vi "Get VI Data.vi"(8 "Error In":errorcluster, 10 "Wik Help Base URL":string="https://www.labviewmakerhub.com/doku.php?id=learn:libraries:linx:reference:labview:", 11 "VI Reference":refnum<vi>) -> (0 "Error Out":errorcluster, 3 "VI Data":T1)   [LabVIEW 2014]
uses:
  VI Data.ctl
  Control Info.ctl
  <vilib>/picture/picture.llb/imagedata.ctl
  <vilib>/Utility/traverseref.llb/TRef TravTarget.ctl
  <vilib>/Utility/traverseref.llb/VI Scripting - Traverse.lvlib
  <vilib>/MakerHub/Toolbox/Private/Front Panel Clean Up/LMH-Front-Panel-Clean-Up.lvlib
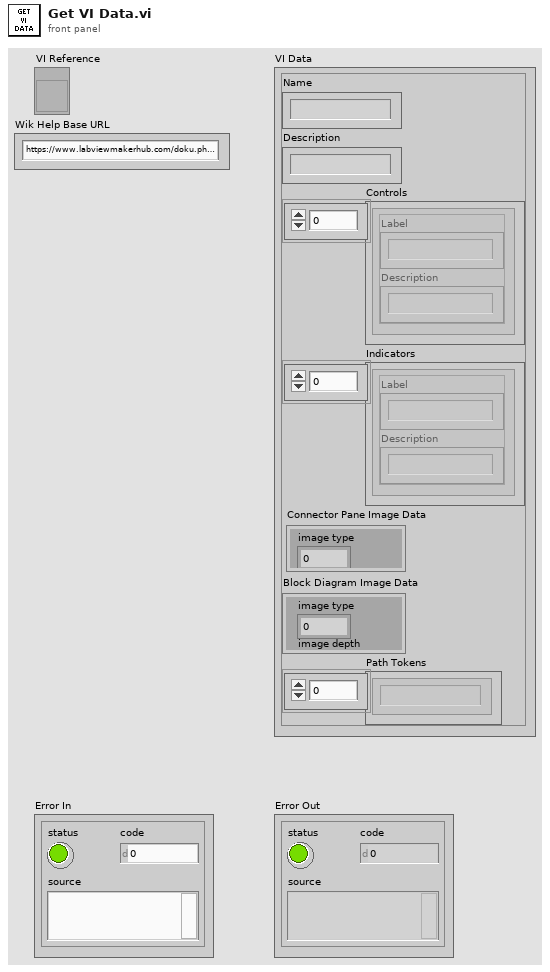
[diagram p1: front panel]
types:
  T1 = typedef "VI Data.ctl" = cluster{"Name":string, "Description":string, "Controls":T2[], "Indicators":T2[], "Connector Pane Image Data":T3, "Block Diagram Image Data":T3, "Path Tokens":string[]}
  T2 = typedef "Control Info.ctl" = cluster{"Label":string, "Description":string}
  T3 = typedef "imagedata.ctl" = cluster{"image type":i32, "image depth":i32, "image":u8[], "mask":u8[], "colors":u32[], "Rectangle":cluster{"left":i16, "top":i16, "right":i16, "bottom":i16}}
  T4 = enum32{"Custom", "Standard", "Using Panel", "Using SubVI", "Complete"}
  T5 = typedef "TRef TravTarget.ctl" = enum16{"FP", "BD", "Other"}
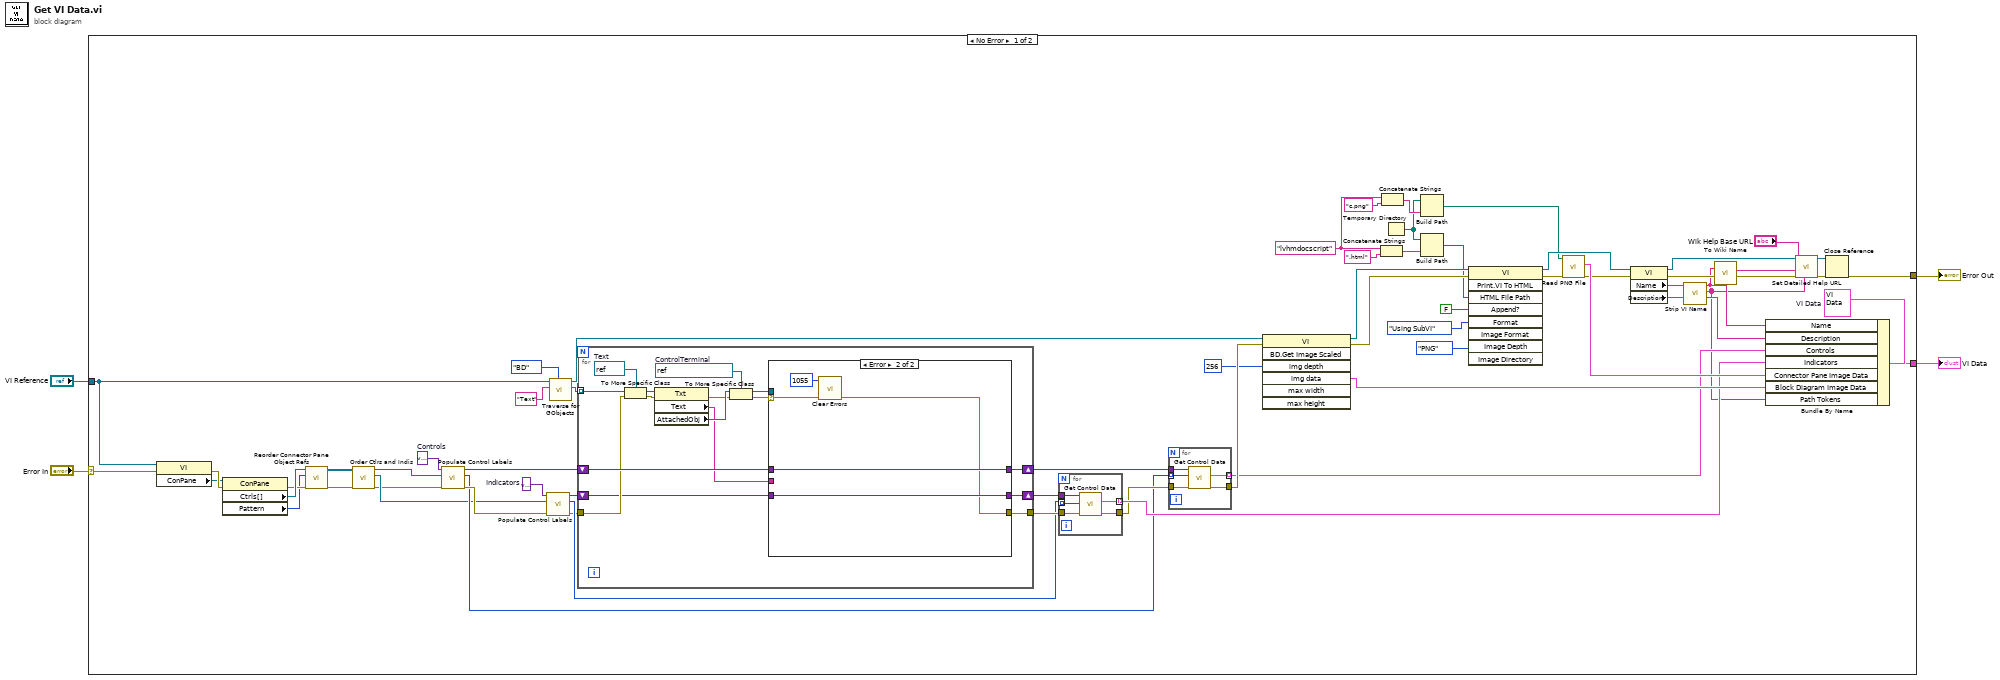
[diagram p0: block diagram]
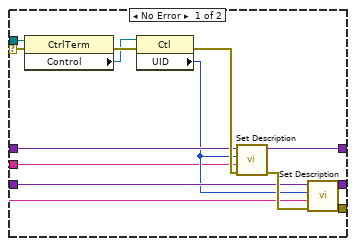
[diagram p2: hidden frame]
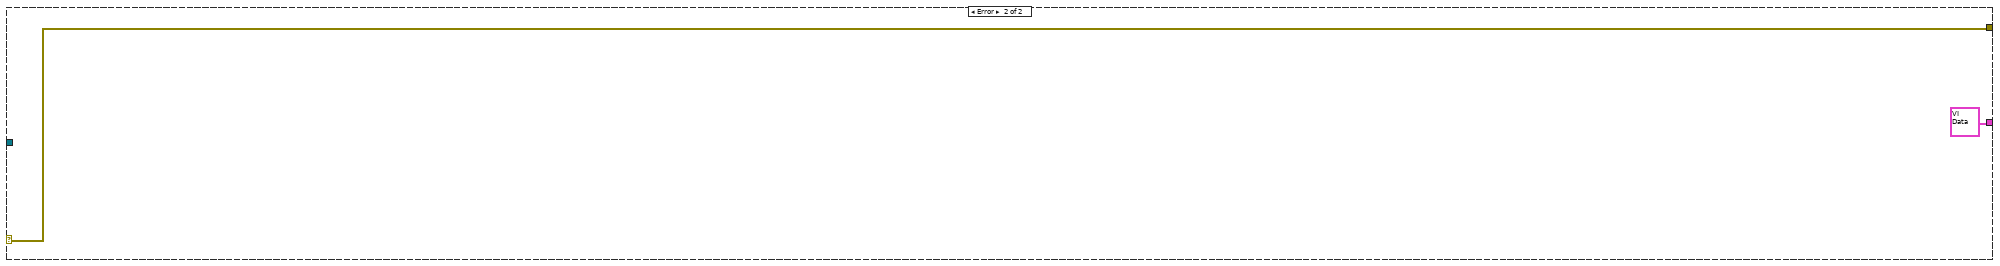
[diagram p3: hidden frame]
diagram:
  n1 = case shown="No Error" "Error In" {
    selector: "Error In" -> [w14 w113]
    tunnel: [w16 T1 {"Name"="", "Description"="", "Controls"=[], "Indicators"=[], "Connector Pane Image Data"={"image type"=0, "image depth"=0, "image"=[], "mask"=[], "colors"=[], "Rectangle"={"left"=0, "top"=0, "right"=0, "bottom"=0}}, "Block Diagram Image Data"={"image type"=0, "image depth"=0, "image"=[], "mask"=[], "colors"=[], "Rectangle"={"left"=0, "top"=0, "right"=0, "bottom"=0}}, "Path Tokens"=[]} ("VI Data")] -> w4
    tunnel: [w12 w113] -> w3
    tunnel: "VI Reference" -> [w15 _]
    frame No Error {
      w17 = T1 {"Name"="", "Description"="", "Controls"=[], "Indicators"=[], "Connector Pane Image Data"={"image type"=0, "image depth"=0, "image"=[], "mask"=[], "colors"=[], "Rectangle"={"left"=0, "top"=0, "right"=0, "bottom"=0}}, "Block Diagram Image Data"={"image type"=0, "image depth"=0, "image"=[], "mask"=[], "colors"=[], "Rectangle"={"left"=0, "top"=0, "right"=0, "bottom"=0}}, "Path Tokens"=[]}  # VI Data
      w57 = "lvhmdocscript" ("string")
      w27 = variant  # Indicators
      w30 = variant  # Controls
      n2 = property class="VI"(reference=w15, error in=w14) -> (error out=w67:errorcluster, "ConPane"=w21:refnum<vi>)  [unwired: 1 out]
      n3 = property class="ConPane"(reference=w21, error in=w67) -> (error out=w23:errorcluster, "Ctrls[]"=w24:refnum<vi>[], "Pattern"=w22:u32)  [unwired: 1 out]
      n4 = call <vilib>:"Reorder Connector Pane Object Refs.vi"("Error In"=w23, "Connector Pane Patter"=w22, "Connector Pane Object Refs"=w24) -> ("Error Out"=w34:errorcluster, "Connector Pane Object Refs"=w25:refnum<vi>[][])  [unwired: 7 in]
      n5 = call "Order Ctlrs and Indis.vi"("Error In"=w34, "Connector Pane Object Refs"=w25) -> ("Error Out"=w28:errorcluster, "Ordered  Indicators"=w29:refnum<vi>[], "Ordered Controls"=w26:refnum<vi>[])  [unwired: 7 in]
      n6 = call "Populate Control Labels.vi"("error in (no error)"=w28, "Ordered Controls"=w26, "Controls in"=w30) -> ("error out"=w35:errorcluster, "UIDs"=w31:i32[], "Controls out"=w33:variant)  [unwired: 6 in]
      n7 = call "Populate Control Labels.vi"("error in (no error)"=w35, "Ordered Controls"=w29, "Controls in"=w27) -> ("error out"=w36:errorcluster, "UIDs"=w39:i32[], "Controls out"=w38:variant)  [unwired: 6 in]
      n8 = call <vilib>:"Traverse for GObjects.vi"("Traverse Target"=TRef_TravTarget."BD", "Class Name"="Text", "VI Refnum"=w15) -> ("References"=w20:refnum<vi>[], "dup VI Refnum"=w47:refnum<vi>)  [unwired: 5 in, 2 out]
      n9 = for {
        tunnel: w20 -> [w92] mode=indexing
        shift-right: [w85] -> w32
        shift-left: w33 -> [w84]
        tunnel: w36 -> [w83]
        shift-right: [w82] -> w37
        shift-left: w38 -> [w81]
        tunnel: [w80] -> w41
        w88 = refnum<vi> refnum  # ControlTerminal
        w93 = refnum<vi> refnum  # Text
        n10 = To More Specific Class(target class=w93, reference=w92, error in=w83) -> (specific class reference=w91:refnum<vi>, error out=w90:errorcluster)
        n11 = property class="Txt"(reference=w91, error in=w90) -> (error out=w86:errorcluster, "Text"=w79:string, "AttachedObj"=w89:refnum<vi>)  [unwired: 1 out]
        n12 = To More Specific Class(target class=w88, reference=w89, error in=w86) -> (specific class reference=w87:refnum<vi>, error out=w78:errorcluster)
        n13 = case shown="Error" w78 {
          selector: w78 -> [w94 w107]
          tunnel: w87 -> [w106 _]
          tunnel: [w102 w110] -> w85
          tunnel: w84 -> [w101 w110]
          tunnel: [w99 w111] -> w82
          tunnel: w81 -> [w98 w111]
          tunnel: [w97 w108] -> w80
          tunnel: w79 -> [w95 _]
          frame No Error {
            n14 = property class="CtrlTerm"(reference=w106, error in=w94) -> (error out=w104:errorcluster, "Control"=w103:refnum<vi>)  [unwired: 1 out]
            n15 = property class="Ctl"(reference=w103, error in=w104) -> (error out=w105:errorcluster, "UID"=w96:i32)  [unwired: 1 out]
            n16 = call "Set Description.vi"("Error In"=w105, "Description"=w95, "UID"=w96, "Controls"=w101) -> ("Error Out"=w100:errorcluster, "Controls"=w102:variant)  [unwired: 6 in]
            n17 = call "Set Description.vi"("Error In"=w100, "Description"=w95, "UID"=w96, "Controls"=w98) -> ("Error Out"=w97:errorcluster, "Controls"=w99:variant)  [unwired: 6 in]
          }
          frame Error {
            n18 = call <vilib>:"Clear Errors.vi"("error in (no error)"=w107, "specific error code to clear (0: all)"=1055) -> ("error out"=w108:errorcluster)  [unwired: 4 in, 1 out]
          }
        }
      }
      n19 = for {
        tunnel: w37 -> [w72]
        tunnel: [w71] -> w40
        tunnel: [w70] -> w44 mode=indexing
        tunnel: w39 -> [w69] mode=indexing
        tunnel: w41 -> [w68]
        n20 = call "Get Control Data.vi"("Error In"=w68, "UID"=w69, "Controls"=w72) -> ("Error Out"=w71:errorcluster, "Control Data"=w70:T2)  [unwired: 6 in, 1 out]
      }
      n21 = for {
        tunnel: w31 -> [w77] mode=indexing
        tunnel: w32 -> [w76]
        tunnel: [w75] -> w46
        tunnel: [w74] -> w43 mode=indexing
        tunnel: w40 -> [w73]
        n22 = call "Get Control Data.vi"("Error In"=w73, "UID"=w77, "Controls"=w76) -> ("Error Out"=w75:errorcluster, "Control Data"=w74:T2)  [unwired: 6 in, 1 out]
      }
      n23 = invoke class="VI" method="BD.Get Image Scaled"(reference=w47, error in=w46, "img depth"=256 ("Image Depth")) -> (reference out=w61:refnum<vi>, error out=w60:errorcluster, "img data"=w66:T3)  [unwired: 4 in, 4 out]
      n24 = Concatenate Strings(w57, ".html" ("name or relative path")) -> (w53:string)
      n25 = Concatenate Strings(w57, "c.png" ("string")) -> (w56:string)
      n26 = Temporary Directory() -> (w54:path)
      n27 = Build Path(base path=w54, name or relative path=w56) -> (appended path=w58:path)
      n28 = Build Path(base path=w54, name or relative path=w53) -> (appended path=w50:path)
      n29 = invoke class="VI" method="Print.VI To HTML"(reference=w61, error in=w60, "HTML File Path"=w50, "Append?"=FALSE, "Format"=T4."Using SubVI", "Image Format"=enum32{"PNG", "JPEG", "GIF"}."PNG") -> (reference out=w63:refnum<vi>, error out=w51:errorcluster)  [unwired: 3 in, 7 out]
      n30 = call <vilib>:"Read PNG File.vi"("error in (no error)"=w51, "path to PNG file"=w58) -> ("error out"=w62:errorcluster, "image data"=w65:T3)  [unwired: 7 in, 1 out]
      n31 = property class="VI"(reference=w63, error in=w62) -> (reference out=w10:refnum<vi>, error out=w9:errorcluster, "Name"=w64:string, "Description"=w42:string)
      n32 = call "Strip VI Name.vi"("Full VI Name"=w64) -> ("Path Tokens"=w6:string[], "Stripped Name"=w8:string)  [unwired: 7 in]
      n33 = call "To Wiki Name.vi"("Name"=w8) -> ("Wiki Name"=w7:string)  [unwired: 2 in]
      n34 = Bundle By Name(cluster=w17, "Name"=w8, "Description"=w42, "Controls"=w43, "Indicators"=w44, "Connector Pane Image Data"=w65, "Block Diagram Image Data"=w66, "Path Tokens"=w6) -> (w16:T1)
      n35 = call "Set Detailed Help URL.vi"("Path Tokens"=w6, "Error In"=w9, "Page Name"=w7, "Wik Help Base URL"="Wik Help Base URL", "VI Refnum"=w10) -> ("Error Out"=w13:errorcluster, "VI Refnum"=w11:refnum<vi>)  [unwired: 5 in]
      n36 = Close Reference(reference=w11, error in (no error)=w13) -> (error out=w12:errorcluster)
    }
    frame Error {
    }
  }
  "Error Out" <- w3
  "VI Data" <- w4
